vi "JamesPIDTEST.vi"() -> ()   [LabVIEW 2014]
uses:
  <vilib>/Rock Robotics/WPI/Solenoid/WPI_SolenoidValue.ctl
  <vilib>/Rock Robotics/WPI/DriverStation/WPI_DriverStationRobotMode2.ctl
  Robot Global Data.vi
  <vilib>/addons/control/pid/pid.llb/PID Advanced (DBL).vi
  <vilib>/addons/control/pid/NI_PID_pid.lvlib
panel:
  out "Setpoint":dbl
  in  "setpoint range":cluster{"setpoint high":dbl, "setpoint low":dbl}={"setpoint high"=100.0, "setpoint low"=0.0}
  out "output":dbl format="%.2f"
  out "Brake":bool
  in  "proportional gain (Kc)":dbl step=0.01
  in  "integral time (Ti, min)":dbl step=0.01
  in  "derivative time (Td, min)":dbl step=0.01
  in  "dt (s)":dbl=-1.0 format="%.3f"
  in  "SetPoint":dbl(slide) scale=3.7..4.5
  out "dx/dt":dbl format="%.3f"
  out "Grabber":bool
  out "Average from Array":dbl
  out "In Range?":bool
  out "Turn on Brake":bool
  out "Delay?":bool
  out "VoltageDiff Valid?":bool
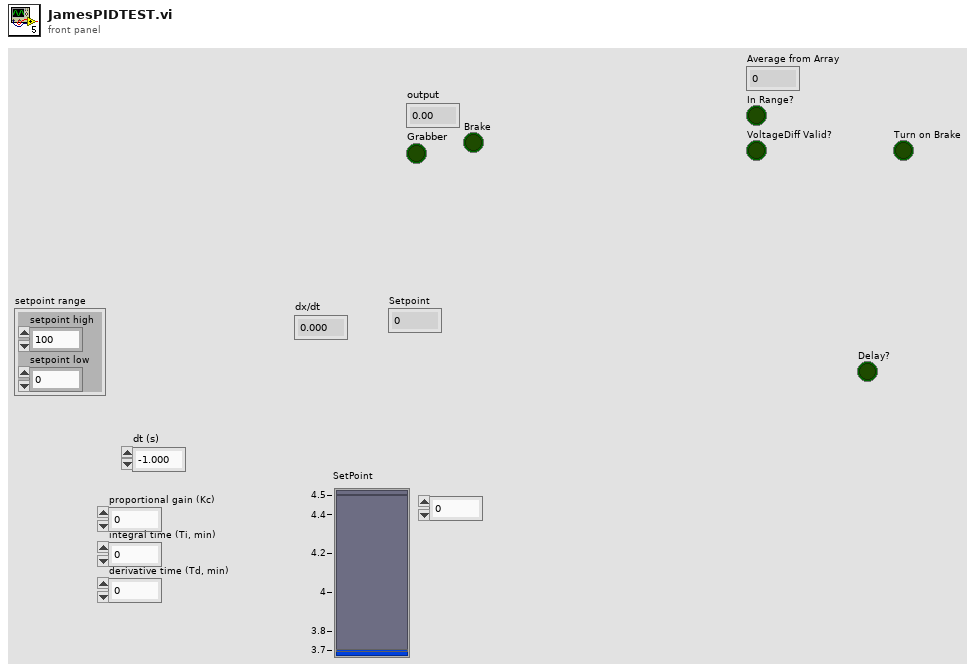
[diagram p1: front panel]
types:
  T1 = typedef "WPI_SolenoidDevRef.ctl" = cluster{"DevStatus":errorcluster, "Pneumatics Control Module":u8, "Forward Solenoid Channel":T2, "Reverse Solenoid Channel":T2}
  T2 = typedef "WPI_SolenoidChannel.ctl" = enum8{"Solenoid 0", "Solenoid 1", "Solenoid 2", "Solenoid 3", "Solenoid 4", "Solenoid 5", "Solenoid 6", "Solenoid 7", "Invalid"}
  T3 = typedef "WPI_MotorControlDeviceRef.ctl" = cluster{"DeviceStatus":errorcluster, "Type":T4, "PWM":cluster{"Controller":T5, "PWM Channel":T6, "DeadBand":T7}, "CAN":cluster{"Device Number":u8, "Control Mode":T8, "Semaphore":T9, "Max Vout":dbl, "TalonSRX Control Mode":T10}, "Invert":bool, "TransformRef":T11, "InvTransformRef":T11}
  T4 = typedef "WPI_MotorControlType.ctl" = enum16{"PWM", "CAN", "CANTalonSRX"}
  T5 = typedef "FPGA_TypedefDigitalModule.ctl" = enum16{"Controller 1"}
  T6 = typedef "FPGA_DIOPWMChannel.ctl" = enum8{"PWM 0", "PWM 1", "PWM 2", "PWM 3", "PWM 4", "PWM 5", "PWM 6", "PWM 7", "PWM 8", "PWM 9", "PWM MXP 0", "PWM MXP 1", "PWM MXP 2", "PWM MXP 3", "PWM MXP 4", "PWM MXP 5", "PWM MXP 6", "PWM MXP 7", "PWM MXP 8", "PWM MXP 9", "Invalid"}
  T7 = typedef "WPI_PWMDeadband.ctl" = cluster{"Name":string, "maxPositivePwm":i32, "minPositivePwm":i32, "centerPwm":i32, "maxNegativePwm":i32, "minNegativePwm":i32, "angularRange":u16}
  T8 = typedef "WPI_CANJaguar_ControlMode.ctl" = enum8{"Percent VBus", "Current", "Speed", "Position", "Voltage"}
  T9 = typedef "Semaphore RefNum" = refnum<k1>
  T10 = typedef "WPI_CANTalonSRX_APIControlMode.ctl" = enum8{"Percent VBus", "Speed", "Position", "Slave", "Unchanged / Invalid"}
  T11 = typedef "WPI_PWMTransform_ConPane.ctl" = refnum<vi>
  T12 = typedef "WPI_SolenoidValue.ctl" = enum16{"Off", "On", "Forward", "Reverse"}
  T13 = typedef "WPI_DriverStationRobotMode2.ctl" = enum16{"Autonomous Disabled", "Autonomous Enabled", "Teleop Disabled", "Teleop Enabled", "Disconnected", "Finish", "Test Disabled", "Test Enabled", "Emergency Stopped"}
  T14 = cluster{"proportional gain (Kc)":dbl, "integral time (Ti, min)":dbl, "derivative time (Td, min)":dbl}
  T15 = cluster{"Motor Speed":dbl, "Grabber":bool, "Brake":bool, "Trying To Brake":bool}
  T16 = cluster{"Front Right Motor":dbl, "Front Left Motor":dbl, "Rear Right Motor":dbl, "Rear Left Motor":dbl, "Current Heading":dbl, "Tote lift Up":bool, "Primary Feeder running":bool, "Secondary Feeder running":bool, "Totes In Robot":dbl, "Pressure In Tank":dbl, "Can Grabber State":T12}
  T17 = cluster{"String Potentiometer":dbl, "Setpoint":dbl, "Level":sgl}
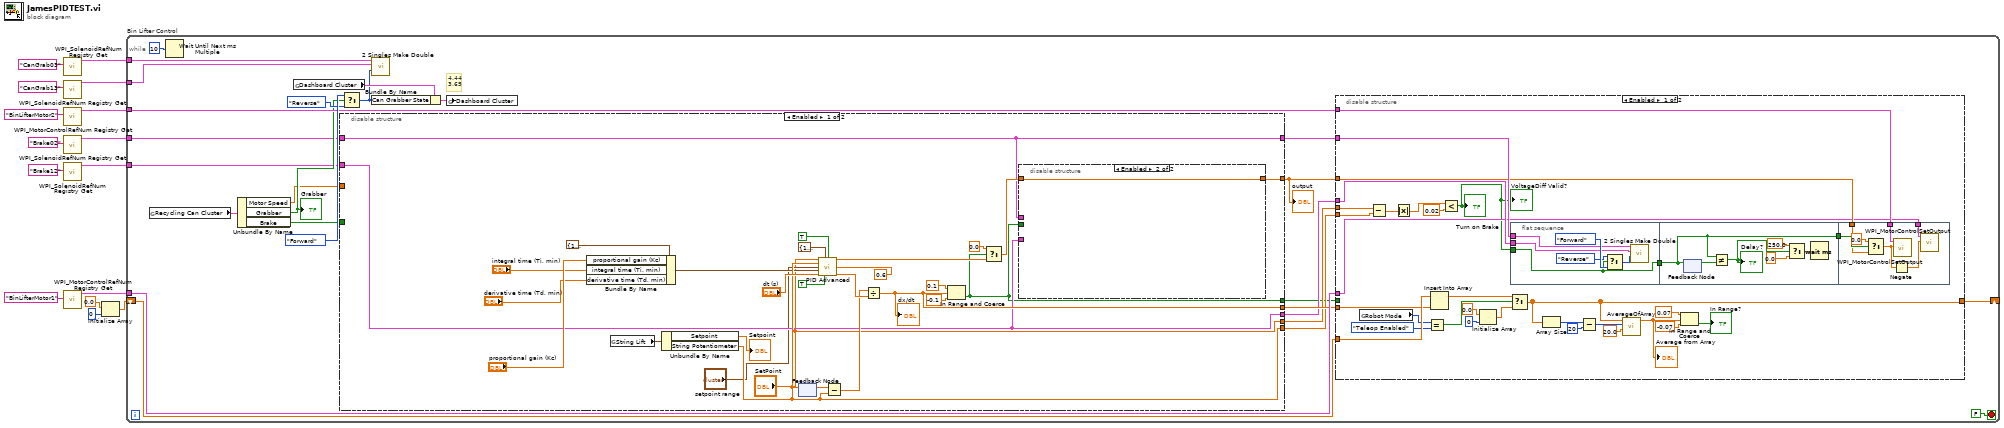
[diagram p0: block diagram]
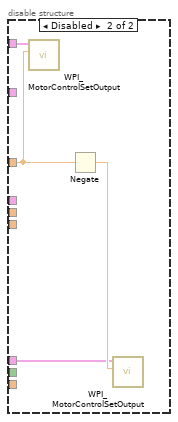
[diagram p2: hidden frame]
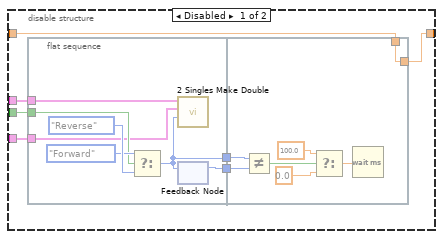
[diagram p3: hidden frame]
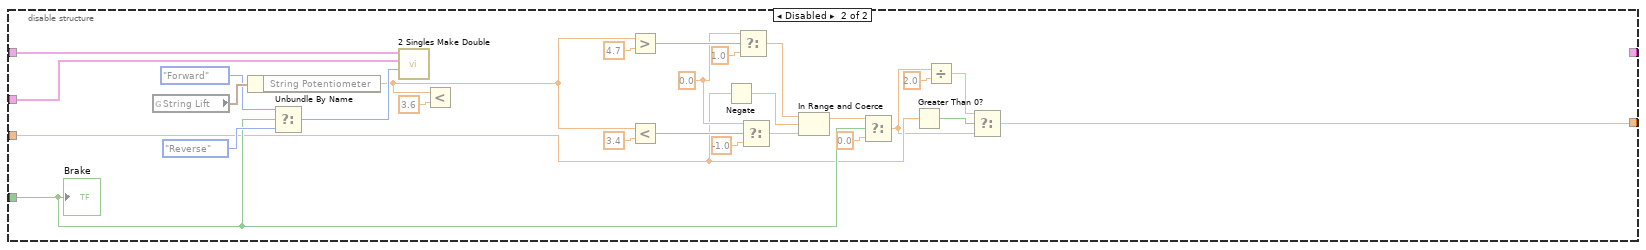
[diagram p4: hidden frame]
diagram:
  n1 = call <vilib>:"WPI_SolenoidRefNum Registry Get.vi"("refnum name"="CanGrab03") -> ("SolenoidDevRef"=w7:T1)  [unwired: 9 in, 1 out]
  n2 = call <vilib>:"WPI_SolenoidRefNum Registry Get.vi"("refnum name"="CanGrab13") -> ("SolenoidDevRef"=w6:T1)  [unwired: 9 in, 1 out]
  n3 = call <vilib>:"WPI_MotorControlRefNum Registry Get.vi"("refnum name"="BinLifterMotor2") -> ("MotorControlDevRef"=w5:T3)  [unwired: 9 in, 1 out]
  n4 = call <vilib>:"WPI_SolenoidRefNum Registry Get.vi"("refnum name"="Brake02") -> ("SolenoidDevRef"=w4:T1)  [unwired: 9 in, 1 out]
  n5 = call <vilib>:"WPI_SolenoidRefNum Registry Get.vi"("refnum name"="Brake12") -> ("SolenoidDevRef"=w3:T1)  [unwired: 9 in, 1 out]
  n6 = call <vilib>:"WPI_MotorControlRefNum Registry Get.vi"("refnum name"="BinLifterMotor1") -> ("MotorControlDevRef"=w2:T3)  [unwired: 9 in, 1 out]
  n7 = Initialize Array(0.0 ("element"), 0 ("dimension size")) -> (w1:dbl[])
  n8 = while "Bin Lifter Control" {
    tunnel: w5 -> [w35]
    tunnel: w2 -> [w34]
    tunnel: w6 -> [w30]
    tunnel: w7 -> [w31]
    tunnel: w4 -> [w26]
    tunnel: w3 -> [w25]
    shift-right: [w22] -> _
    shift-left: w1 -> [w24]
    stop <- FALSE stop-if-true
    # "4.44\n3.65"
    n9 = global read "Robot Global Data.vi" "Recycling Can Cluster"() -> (w40:T15)
    n10 = Wait Until Next ms Multiple(millisecond multiple=u32 10) -> ()  [unwired: 1 out]
    n11 = Unbundle By Name(w40) -> ("Motor Speed"=w28:dbl, "Grabber"=w32:bool, "Brake"=w27:bool)
    "Grabber" <- w32
    n12 = global read "Robot Global Data.vi" "Dashboard Cluster"() -> (w36:T16)
    n13 = disable-structure shown="Enabled" {
      disable-tunnel: [w108 w148] -> w19
      disable-tunnel: w28 -> [_ w151]
      disable-tunnel: w27 -> [_ w156]
      disable-tunnel: w26 -> [w105 w158]
      disable-tunnel: w25 -> [w104 w157]
      disable-tunnel: [w107 _] -> w23
      disable-tunnel: ["SetPoint" _] -> w21
      disable-tunnel: [w106 _] -> w20
      disable-tunnel: [w105 _] -> w18
      disable-tunnel: [w104 _] -> w17
      disable-tunnel: [w103 _] -> w16
      frame Enabled {
        n14 = Bundle By Name(cluster=T14 {"proportional gain (Kc)"=1.0, "integral time (Ti, min)"=0.01, "derivative time (Td, min)"=0.0} ("PID gains"), "proportional gain (Kc)"="proportional gain (Kc)", "integral time (Ti, min)"="integral time (Ti, min)", "derivative time (Td, min)"="derivative time (Td, min)") -> (w102:T14)
        n15 = global read "Robot Global Data.vi" "String Lift"() -> (w117:T17)
        n16 = Unbundle By Name(w117) -> ("Setpoint"=→"Setpoint":dbl, "String Potentiometer"=w106:dbl)
        n17 = feedback-in #1(w106) -> ()
        n18 = feedback #1() -> (w116:dbl)  [unwired: 1 in]
        n19 = call-poly <vilib>:"PID Advanced.vi"("setpoint"="SetPoint", "output range"=cluster{"output high":dbl, "output low":dbl} {"output high"=1.0, "output low"=-1.0}, "auto? (T)"=TRUE, "process variable"=w106, "setpoint range"="setpoint range", "alpha"=0.6, "PID gains"=w102, "dt (s)"="dt (s)", "reinitialize? (F)"=TRUE ("autotune? (F)")) -> ("output"=w111:dbl, "dt out (s)"=w115:dbl)  [unwired: 5 in]
        n20 = Subtract(x=w116, y=w106) -> (x-y=w114:dbl)
        n21 = Divide(x=w114, y=w115) -> (x/y=w107:dbl)
        "dx/dt" <- w107
        n22 = In Range and Coerce(upper limit=0.1, x=w107, lower limit=-0.1) -> (In Range?=w103:bool)  [unwired: 1 out]
        n23 = Select(t=0.0, s=w103, f=w111) -> (s? t:f=w109:dbl)
        n24 = disable-structure shown="Enabled" {
          disable-tunnel: w103 -> [w128 _]
          disable-tunnel: w105 -> [w127 _]
          disable-tunnel: w104 -> [w126 _]
          disable-tunnel: w109 -> [w125 w145]
          disable-tunnel: [w124 w145] -> w108
          frame Disabled {
            n25 = flat-sequence {
              tunnel: w128 -> [w135]
              tunnel: w127 -> [w134]
              tunnel: w126 -> [w133]
              tunnel: [w132] -> w130
              tunnel: [w131] -> w129
              tunnel: w125 -> [w144]
              tunnel: [w144] -> w124
              tunnel: w130 -> [w143]
              tunnel: w129 -> [w142]
              frame #0 {
                n26 = Select(t=WPI_SolenoidValue."Forward" ("Value"), s=w135, f=WPI_SolenoidValue."Reverse" ("Value")) -> (s? t:f=w132:T12)
                n27 = call "2 Singles Make Double.vi"("Value"=w132, "Reverse In"=w133, "Forward In"=w134) -> ()  [unwired: 7 in, 2 out]
                n28 = feedback-in #2(w132) -> ()
                n29 = feedback #2() -> (w131:T12)  [unwired: 1 in]
              }
              frame #1 {
                n30 = Not Equal?(x=w143, y=w142) -> (x != y?=w141:bool)
                n31 = Select(t=100.0, s=w141, f=0.0) -> (s? t:f=w140:dbl)
                n32 = Wait (ms)(milliseconds to wait=w140) -> ()  [unwired: 1 out]
              }
            }
          }
          frame Enabled {
          }
        }
      }
      frame Disabled {
        w164 = 0.0 ("t")
        n33 = global read "Robot Global Data.vi" "String Lift"() -> (w172:T17)
        n34 = Unbundle By Name(w172) -> ("String Potentiometer"=w154:dbl)
        n35 = Select(t=WPI_SolenoidValue."Forward" ("Value"), s=w156, f=WPI_SolenoidValue."Reverse" ("Value")) -> (s? t:f=w159:T12)
        n36 = call "2 Singles Make Double.vi"("Value"=w159, "Reverse In"=w157, "Forward In"=w158) -> ()  [unwired: 7 in, 2 out]
        n37 = Less?(x=w154, y=3.6) -> ()  [unwired: 1 out]
        n38 = Greater?(x=w154, y=4.7) -> (0:w169:bool)
        n39 = Less?(x=w154, y=3.4) -> (x < y?=w166:bool)
        n40 = Negate(x=w151) -> (-x=w162:dbl)
        n41 = Select(t=w164, s=w169, f=1.0) -> (s? t:f=w168:dbl)
        n42 = Select(t=w164, s=w166, f=-1.0) -> (s? t:f=w167:dbl)
        n43 = In Range and Coerce(upper limit=w168, x=w162, lower limit=w167) -> (coerced(x)=w147:dbl)  [unwired: 1 out]
        n44 = Select(t=w147, s=w156, f=0.0 ("t")) -> (s? t:f=w150:dbl)
        n45 = Greater Than 0?(x=w151) -> (x > 0?=w153:bool)
        n46 = Divide(x=w150, y=2.0) -> (x/y=w152:dbl)
        n47 = Select(t=w152, s=w153, f=w150) -> (s? t:f=w148:dbl)
        "Brake" <- w156
      }
    }
    "output" <- w19
    n48 = Select(t=WPI_SolenoidValue."Forward" ("Value"), s=w32, f=WPI_SolenoidValue."Reverse" ("Value")) -> (s? t:f=w29:T12)
    n49 = call "2 Singles Make Double.vi"("Value"=w29, "Reverse In"=w30, "Forward In"=w31) -> ()  [unwired: 7 in, 2 out]
    n50 = Bundle By Name(cluster=w36, "Can Grabber State"=w29) -> (w37:T16)
    n51 = global write "Robot Global Data.vi" "Dashboard Cluster"(w37) -> ()
    n52 = disable-structure shown="Enabled" {
      disable-tunnel: w35 -> [w46 w93]
      disable-tunnel: w34 -> [w43 w94]
      disable-tunnel: w24 -> [w72 _]
      disable-tunnel: w23 -> [w71 _]
      disable-tunnel: [w62 _] -> w22
      disable-tunnel: w21 -> [w55 _]
      disable-tunnel: w20 -> [w54 _]
      disable-tunnel: w19 -> [w44 w92]
      disable-tunnel: w18 -> [w50 _]
      disable-tunnel: w17 -> [w49 _]
      disable-tunnel: w16 -> [_ _]
      frame Enabled {
        n53 = global read "Robot Global Data.vi" "Robot Mode"() -> (w70:T13)
        n54 = Subtract(x=w55, y=w54) -> (x-y=w53:dbl)
        n55 = Absolute Value(x=w53) -> (abs(x)=w52:dbl)
        n56 = Equal?(x=w70, y=WPI_DriverStationRobotMode2."Teleop Enabled") -> (x = y?=w68:bool)
        n57 = Insert Into Array(array=w72, new element=w71) -> (w67:dbl[])  [unwired: 1 in]
        n58 = Less?(x=w52, y=0.02) -> (x < y?=w42:bool)
        "Turn on Brake" <- w42
        "VoltageDiff Valid?" <- w42
        n59 = Initialize Array(0.0 ("element"), 0 ("dimension size")) -> (w64:dbl[])
        n60 = Select(t=w67, s=w68, f=w64) -> (s? t:f=w62:dbl[])
        n61 = flat-sequence {
          tunnel: w42 -> [w73]
          tunnel: w50 -> [w76]
          tunnel: w49 -> [w75]
          tunnel: [w73] -> w47
          tunnel: w47 -> [w79]
          tunnel: [w79] -> w45
          tunnel: w46 -> [w91]
          tunnel: w45 -> [w89]
          tunnel: w44 -> [w88]
          tunnel: w43 -> [w85]
          frame #0 {
            n62 = Select(t=WPI_SolenoidValue."Reverse" ("Value"), s=w73, f=WPI_SolenoidValue."Forward" ("Value")) -> (s? t:f=w74:T12)
            n63 = call "2 Singles Make Double.vi"("Value"=w74, "Reverse In"=w75, "Forward In"=w76) -> ()  [unwired: 7 in, 2 out]
          }
          frame #1 {
            n64 = feedback #3() -> (w80:bool)  [unwired: 1 in]
            n65 = feedback-in #3(w79) -> ()
            n66 = Not Equal?(x=w79, y=w80) -> (x != y?=w84:bool)
            "Delay?" <- w84
            n67 = Select(t=250.0, s=w84, f=0.0) -> (s? t:f=w83:dbl)
            n68 = Wait (ms)(milliseconds to wait=w83) -> ()  [unwired: 1 out]
          }
          frame #2 {
            n69 = Select(t=0.0, s=w89, f=w88) -> (s? t:f=w86:dbl)
            n70 = Negate(x=w86) -> (-x=w87:dbl)
            n71 = call <vilib>:"WPI_MotorControlSetOutput.vi"("Output"=w86, "MotorControlDevRef"=w91) -> ()  [unwired: 7 in, 3 out]
            n72 = call <vilib>:"WPI_MotorControlSetOutput.vi"("Output"=w87, "MotorControlDevRef"=w85) -> ()  [unwired: 7 in, 3 out]
          }
        }
        n73 = Array Size(array=w62) -> (size(s)=w61:i32)
        n74 = Subtract(x=w61, y=20) -> (x-y=w59:i32)
        n75 = call "AverageOfArray.vi"("Length of Sample"=20.0, "Start Index"=w59, "Array In"=w62) -> ("Average"=w58:dbl)  [unwired: 8 in]
        "Average from Array" <- w58
        n76 = In Range and Coerce(upper limit=0.07, x=w58, lower limit=-0.07) -> (In Range?=→"In Range?":bool)  [unwired: 1 out]
      }
      frame Disabled {
        n77 = call <vilib>:"WPI_MotorControlSetOutput.vi"("Output"=w92, "MotorControlDevRef"=w93) -> ()  [unwired: 7 in, 3 out]
        n78 = Negate(x=w92) -> (-x=w95:dbl)
        n79 = call <vilib>:"WPI_MotorControlSetOutput.vi"("Output"=w95, "MotorControlDevRef"=w94) -> ()  [unwired: 7 in, 3 out]
      }
    }
  }
